vi "runHTMLHist.vi"() -> ()   [LabVIEW 2012]
uses:
  <vilib>/Utility/file.llb/Read From Spreadsheet File (string).vi
panel:
  out "element":string
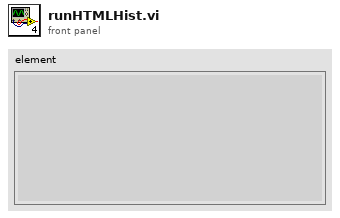
[diagram p1: front panel]
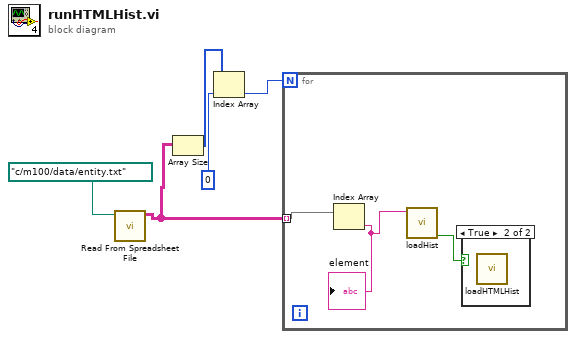
[diagram p0: block diagram]
diagram:
  n1 = call-poly <vilib>:"Read From Spreadsheet File.vi"("file path (dialog if empty)"=path "c:/m100/data/entity.txt" ("file path (use dialog)")) -> ("all rows"=w1:string[][])  [unwired: 6 in, 4 out]
  n2 = Array Size(array=w1) -> (size(s)=w4:i32[])
  n3 = Index Array(array=w4, index=0) -> (element=w2:i32)
  n4 = for {
    N: w2 -> [_]
    tunnel: w1 -> [w8] mode=indexing
    n5 = Index Array(array=w8) -> (element=w7:string)  [unwired: 1 in]
    "element" <- w7
    n6 = call "loadHist.vi"("folder"=w7) -> ("f"=w6:bool)  [unwired: 10 in]
    n7 = case shown="True" w6 {
      frame False {
      }
      frame True {
        n8 = call "loadHTMLHist.vi"() -> ()  [unwired: 12 in]
      }
    }
  }
